vi "Get DAQ Readout Samples.vi"(8 "error in":errorcluster, 11 "INL PID in":refnum<class "INL PID.lvclass">) -> (0 "error out":errorcluster, 2 "ReadOut Samples":i32, 3 "INL PID out":refnum<class "INL PID.lvclass">)   [LabVIEW 2011, in "INL PID.lvclass"]
uses:
  INL PID.lvclass
  INL PID.lvclass/INL PID.ctl
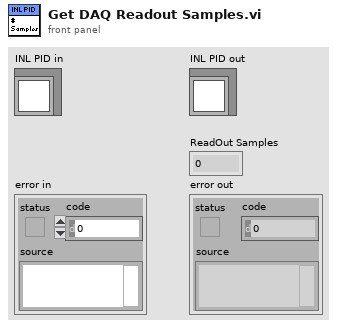
[diagram p1: front panel]
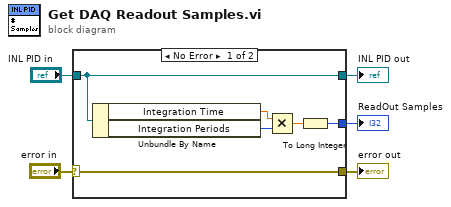
[diagram p0: block diagram]
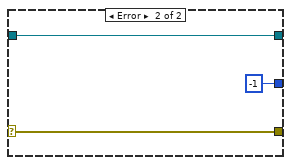
[diagram p2: hidden frame]
diagram:
  n1 = case shown="No Error" "error in" {
    selector: "error in" -> [w11 w14]
    tunnel: [w11 w14] -> w4
    tunnel: [w10 w13] -> w2
    tunnel: "INL PID in" -> [w10 w13]
    tunnel: [w6 -1] -> w1
    frame No Error {
      n2 = Unbundle By Name(w10) -> ("Integration Time"=w8:dbl, "Integration Periods"=w9:u8)
      n3 = Multiply(x=w8, y=w9) -> (x*y=w7:dbl)
      n4 = To Long Integer(number=w7) -> (32bit integer=w6:i32)
    }
    frame Error {
    }
  }
  "error out" <- w4
  "INL PID out" <- w2
  "ReadOut Samples" <- w1
